vi "Read configuration.vi"(7 "force loading?":bool=TRUE, 8 "error in (no error)":errorcluster, 11 "ImageStack in":refnum<class "ImageStack.lvclass">) -> (0 "error out":errorcluster, 3 "ImageStack out":refnum<class "ImageStack.lvclass">)   [LabVIEW 2012]
doc: "Reads the XML-based configuration file and populates the configuration cluster accordingly. Configuration file name is <component ID>.xml."
uses:
  ImageStack.lvclass
  <vilib>/Distrio/Murmex/Murmex/Murmex.lvclass
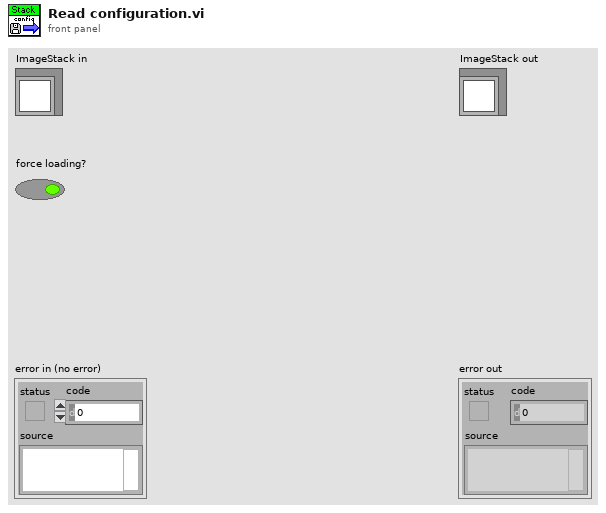
[diagram p1: front panel]
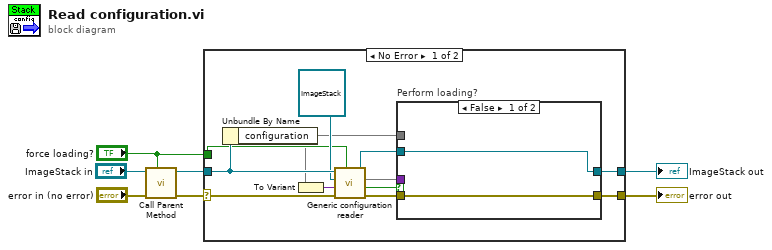
[diagram p0: block diagram]
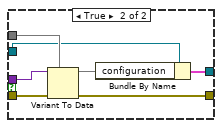
[diagram p2: hidden frame]
diagram:
  n1 = call-parent "Call Parent Method"("force loading?"="force loading?", "error in (no error)"="error in (no error)", "Murmex in"="ImageStack in") -> ("error out"=w5:errorcluster, "Murmex out"=w3:refnum<class "ImageStack.lvclass">)  [unwired: 7 in]
  n2 = case shown="No Error" w5 {
    selector: w5 -> [w19 w29]
    tunnel: [w9 w30] -> w4
    tunnel: w3 -> [w18 w30]
    tunnel: [w8 w29] -> w2
    tunnel: "force loading?" -> [w15 _]
    frame No Error {
      n3 = Unbundle By Name(w18) -> ("configuration"=w11)
      n4 = To Variant(anything=w11) -> (Variant=w17:variant)
      n5 = call <vilib>:"Generic configuration reader.vi"(7:w15, "error in (no error)"=w19, 9:w17, 10:refnum<class "ImageStack.lvclass"> refnum ("ImageStack"), "Murmex in"=w18) -> ("error out"=w13:errorcluster, "loaded?"=w14:bool, 2:w12, "Murmex out"=w10:refnum<class "ImageStack.lvclass">)  [unwired: 3 in]
      n6 = case "Perform loading?" shown="False" w14 {
        tunnel: w13 -> [w21 w28]
        tunnel: w12 -> [_ w27]
        tunnel: w11 -> [_ w26]
        tunnel: w10 -> [w20 w25]
        tunnel: [w20 w23] -> w9
        tunnel: [w21 w22] -> w8
        frame False {
        }
        frame True {
          n7 = Variant To Data(error in=w28, type=w26, Variant=w27) -> (data=w24, error out=w22:errorcluster)
          n8 = Bundle By Name(cluster=w25, "configuration"=w24) -> (w23:cluster{})
        }
      }
    }
    frame Error {
    }
  }
  "error out" <- w2
  "ImageStack out" <- w4
